vi "Split myDAQ Function Select.vi"(0 "IN 7:0":u8 format="%08b") -> (3 "OUT 0":bool, 4 "OUT 1":bool, 5 "OUT 2":bool, 6 "OUT 3":bool)   [LabVIEW 2019]
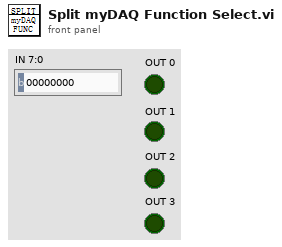
[diagram p1: front panel]
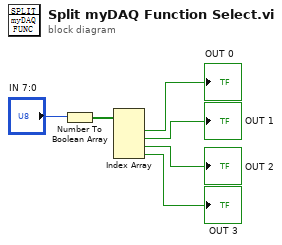
[diagram p0: block diagram]
diagram:
  n1 = Number To Boolean Array(number="IN 7:0") -> (Boolean array=w5:bool[])
  n2 = Index Array(array=w5) -> (element #1=→"OUT 0":bool, element #2=→"OUT 1":bool, element #3=→"OUT 2":bool, element #4=→"OUT 3":bool)  [unwired: 4 in]
